vi "Copy Class Item.vi"(8 "error in (no error)":errorcluster, 9 "New Name":string, 10 "Full path in":path, 11 "LVClassLibrary in":refnum<vi>) -> (0 "error out":errorcluster, 2 "New Class Path out":path, 3 "LVClassLibrary out":refnum<vi>)   [LabVIEW 2019, in "gRPC Template Creation Utility.lvlib"]
uses:
  gRPC Template Creation Utility.lvlib
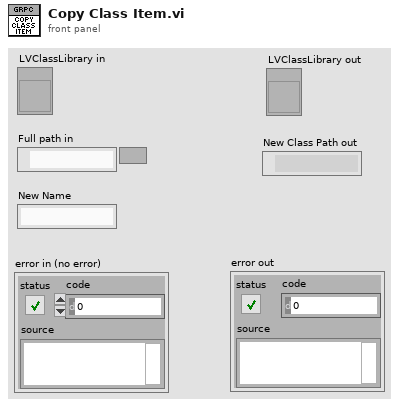
[diagram p1: front panel]
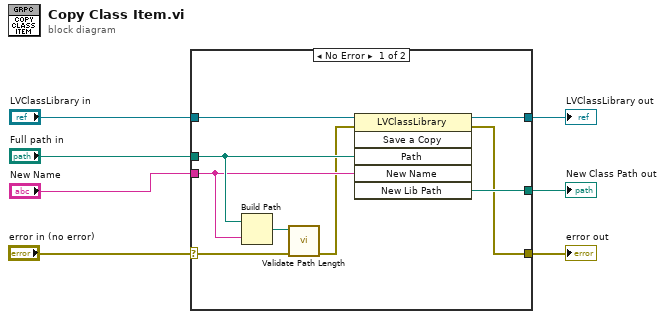
[diagram p0: block diagram]
diagram:
  n1 = case shown="No Error" "error in (no error)" {
    selector: "error in (no error)" -> [w14 w18]
    tunnel: [w16 _] -> w7
    tunnel: "New Name" -> [w10 _]
    tunnel: "Full path in" -> [w11 _]
    tunnel: "LVClassLibrary in" -> [w15 w17]
    tunnel: [w13 w18] -> w2
    tunnel: [w12 w17] -> w1
    frame No Error {
      n2 = Build Path(base path=w11, name or relative path=w10) -> (appended path=w8:path)
      n3 = call "Validate Path Length.vi"("error in (no error)"=w14, "Path in"=w8) -> ("error out"=w9:errorcluster)  [unwired: 8 in, 1 out]
      n4 = invoke class="LVClassLibrary" method="Save a Copy"(reference=w15, error in=w9, "Path"=w11, "New Name"=w10) -> (reference out=w12:refnum<vi>, error out=w13:errorcluster, "New Lib Path"=w16:path)  [unwired: 2 in, 3 out]
    }
    frame Error {
    }
  }
  "New Class Path out" <- w7
  "error out" <- w2
  "LVClassLibrary out" <- w1
